vi "Close.vi"(8 "Error In":errorcluster, 11 "reference in":refnum<class "Camera.lvclass">) -> (0 "Error Out":errorcluster, 3 "reference out":refnum<class "Camera.lvclass">)   [LabVIEW 2025, in "Camera.lvclass"]
uses:
  Camera.lvclass
  Interfaces/IConfigure/IConfigure.lvclass
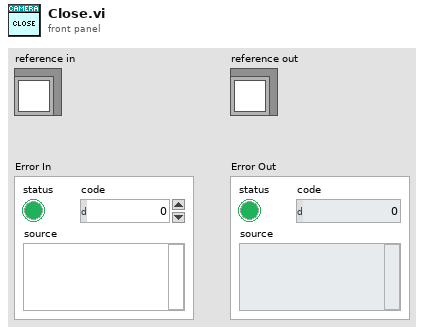
[diagram p1: front panel]
types:
  T1 = typedef "Camera.lvclass/ObjectAttributes.ctl" = cluster{"IConfigure":refnum<class "IConfigure.lvclass">, "Worker Enqueuer":refnum<class "Message Enqueuer.lvclass">, "Start Counter":i32, "Initialized":bool}
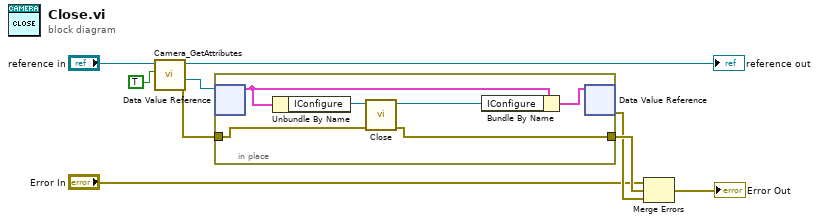
[diagram p0: block diagram]
diagram:
  n1 = call "Camera_GetAttributes.vi"("OnlyGetDvrReference(False)"=TRUE, "reference in"="reference in") -> ("Error Out"=w4:errorcluster, "DataRef"=w3:refnum<data-value>, "reference out"=→"reference out":refnum<class "Camera.lvclass">)  [unwired: 6 in, 1 out]
  n2 = in-place {
    in-place-border: w4 -> [w14]
    in-place-border: [w13] -> w6
    n3 = in-place-dvr #1(w3) -> (w12:T1)  [unwired: 1 out]
    n4 = Unbundle By Name(w12) -> ("IConfigure"=w15:refnum<class "IConfigure.lvclass">)
    n5 = call-dynamic "Close.vi"("error in"=w14, "IClose in"=w15) -> ("error out"=w13:errorcluster, "IClose out"=w11:refnum<class "IConfigure.lvclass">)  [unwired: 8 in]
    n6 = Bundle By Name(cluster=w12, "IConfigure"=w11) -> (w10:T1)
    n7 = in-place-dvr #1(w10) -> (w2:errorcluster)  [unwired: 1 out]
  }
  n8 = Merge Errors("Error In", w6, w2) -> (→"Error Out":errorcluster)
